vi "Unstylized UI - After LSS has been run.vi"() -> ()   [LabVIEW 2019, in "LSS.lvlib"]
doc: "This example demonstrates the application of LSS properties to a wide variety of front panel controls. The \"UI With No Styles.vi\" is what the VI looks like before application of styles, and the \"UI With No Styles - Modified.vi\" shows what the application looks like after the application of a single style sheet with many definitions."
uses:
  LSS.lvlib
panel:
  in  "STOP":bool
  in  "Enum":enum16{"Test", "Test2"}(ring)
  in  "Color Box":u32(colorbox)
  in  "Knob":dbl(knob) scale=0.0..10.0
  in  "Array":dbl[][](array[numeric])
  in  "Tab Control":enum32{"Page 1", "Page 2"}(tab)
  in  "OK Button":bool
  in  "Boolean 3":bool
  in  "Radio Buttons":enum32{"Radio Selection 1", "Radio Selection 2"}(radio)
  in  "Slide":dbl(slide) scale=0.0..10.0
  in  "Switch":bool
  out "Waveform Chart":dbl(graph)
  out "LED":bool
  in  "Num":dbl
  out "error out":errorcluster
  out "PathIndicator":path
  in  "PathControl":path
  in  "Combo Box":string(combo)
  in  "StringControl":string
  out "StringIndicator":string
  out "SquareLED":bool
  in  "Ring":u16(ring) items=["Test", "Test2"]
  # "This is a free label"
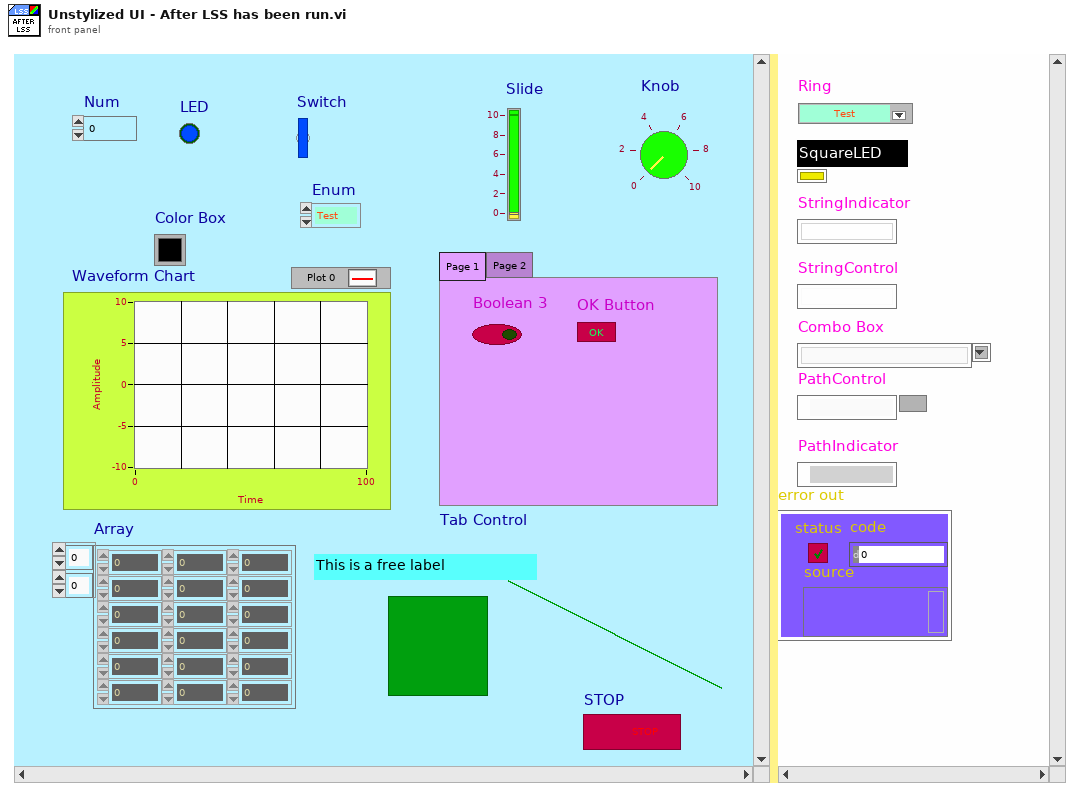
[diagram p1: front panel]
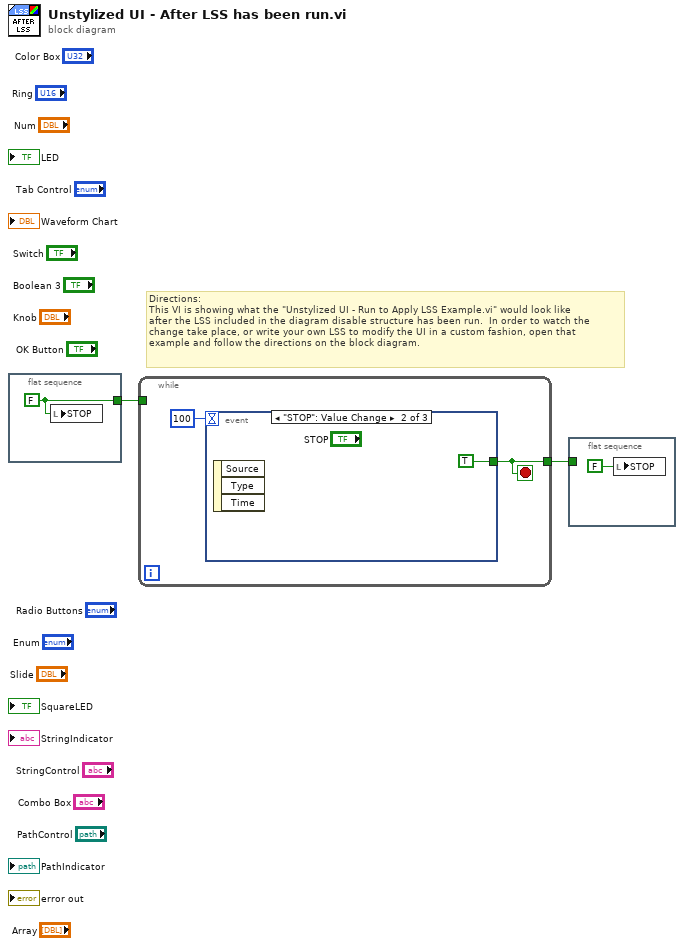
[diagram p0: block diagram]
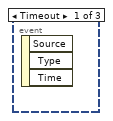
[diagram p2: hidden frame]
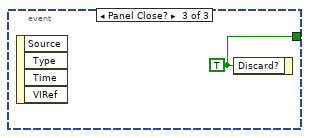
[diagram p3: hidden frame]
diagram:
  # "Directions:\nThis VI is showing what the \"Unstylized UI - Run to Apply LSS Example.vi\" would look like\nafter the LSS included in the diagram disable structure has been run.  In order to watch the\nchange take place, or write your own LSS to modify the UI in a custom fashion, open that\nexample and follow the directions on the block diagram."
  n1 = flat-sequence {
    tunnel: [w3] -> w2
    frame #0 {
      w3 = FALSE ("STOP")
      n2 = local write "STOP"(w3) -> ()
    }
  }
  n3 = while {
    tunnel: w2 -> [_]
    tunnel: [w4] -> w1
    stop <- w4 stop-if-true
    n4 = event shown="[1] \"STOP\": Value Change" {
      selector: _ -> [_ _ _]
      dyn-events: _ -> [_ _ _]
      timeout: u32 100 ("milliseconds to wait") -> [_ _ _]
      tunnel: [_ TRUE w7] -> w4
      event Timeout {
        n5 = event-data() -> ()  [unwired: 1 in, 3 out]
      }
      event "STOP": Value Change {
        n6 = event-data() -> ()  [unwired: 1 in, 3 out]
      }
      event Panel Close? {
        w7 = TRUE ("Discard?")
        n7 = event-data() -> ()  [unwired: 1 in, 4 out]
        n8 = event-data("Discard?"=w7) -> ()  [unwired: 1 in, 1 out]
      }
    }
  }
  n9 = flat-sequence {
    tunnel: w1 -> [_]
    frame #0 {
      n10 = local write "STOP"(FALSE ("STOP")) -> ()
    }
  }
